vi "layout.vi"(0 "reference":refnum<class "StateNode.lvclass">, 1 "graph":refnum<class "Graph.lvclass">, 2 "graphics":refnum<class "Graphics.lvclass">, 3 "grid":refnum<class "Grid.lvclass">, 5 "error in (no error)":errorcluster) -> (14 "reference out":refnum<class "StateNode.lvclass">, 19 "error out":errorcluster)   [LabVIEW 2014, in "StateNode.lvclass"]
doc: "public void layout(Graph g, Graphics2D g2, Grid grid)"
uses:
  <resource>/Framework/Providers/Open_GDS/UML/StateNode_class/StateNode.lvclass
  <resource>/Framework/Providers/Open_GDS/UML/Graph_class/Graph.lvclass
  <resource>/Framework/Providers/Open_GDS/UML/Graphics_class/Graphics.lvclass
  <resource>/Framework/Providers/Open_GDS/UML/Grid_class/Grid.lvclass
  <resource>/Framework/Providers/Open_GDS/UML/General/Rectangle/Rectangle Rectangle2D.ctl
  <resource>/Framework/Providers/Open_GDS/UML/MultiLineString_class/MultiLineString.lvclass
  <resource>/Framework/Providers/Open_GDS/UML/RectangularNode_class/RectangularNode.lvclass
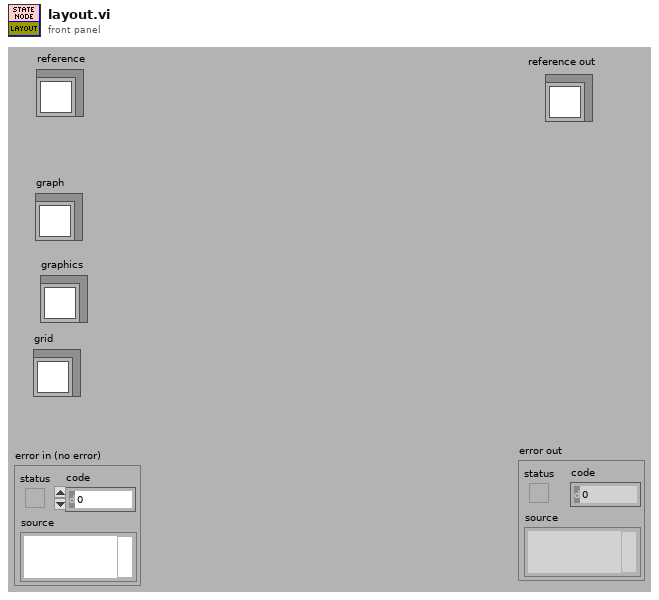
[diagram p1: front panel]
types:
  T1 = typedef "Rectangle Rectangle2D.ctl" = cluster{"x":dbl, "y":dbl, "width":dbl, "height":dbl}
  T2 = typedef "StateNode.lvclass/ObjectAttributes.ctl" = cluster{"state":refnum<class "MultiLineString.lvclass">, "action":refnum<class "MultiLineString.lvclass">, "DEFAULT_WIDTH":i32, "DEFAULT_HEIGHT":i32}
  T3 = typedef "RectangularNode.lvclass/ObjectAttributes.ctl" = cluster{"bounds":T1}
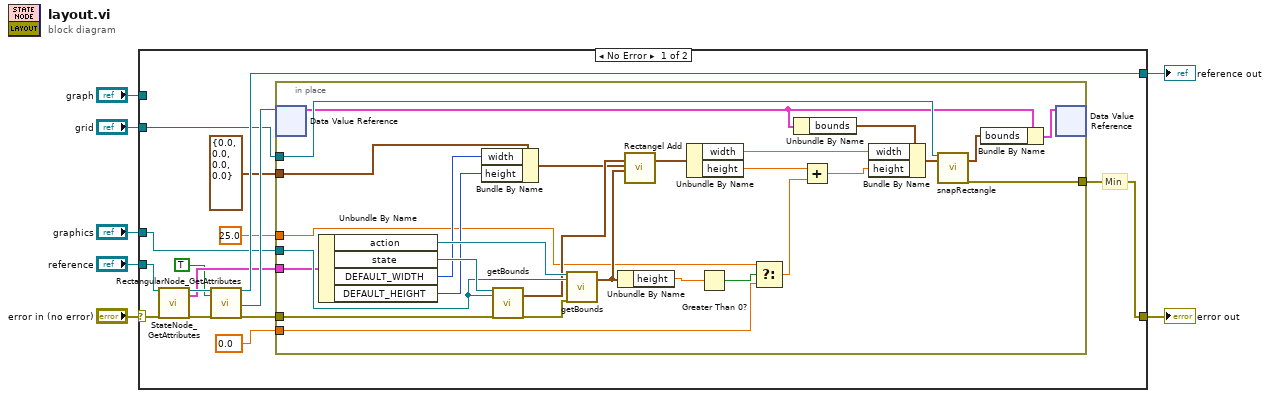
[diagram p0: block diagram]
diagram:
  n1 = case shown="No Error" "error in (no error)" {
    selector: "error in (no error)" -> [w20 w51]
    tunnel: "reference" -> [w22 w52]
    tunnel: [w10 w51] -> w6
    tunnel: [w21 w52] -> w5
    tunnel: "graph" -> [_ _]
    tunnel: "graphics" -> [w16 _]
    tunnel: "grid" -> [w11 _]
    frame No Error {
      # "Min"
      n2 = call <resource>:"StateNode_GetAttributes.vi"("reference in"=w22, "error in (no error)"=w20) -> ("reference out"=w19:refnum<class "StateNode.lvclass">, "Data"=w9:T2, "error out"=w18:errorcluster)  [unwired: 14 in, 1 out]
      n3 = call <resource>:"RectangularNode_GetAttributes.vi"("reference in"=w19, "OnlyGetDvrReference(False)"=TRUE, "error in (no error)"=w18) -> ("reference out"=w21:refnum<class "StateNode.lvclass">, "DataRef"=w17:refnum<data-value>, "error out"=w15:errorcluster)  [unwired: 13 in, 1 out]
      n4 = in-place {
        in-place-border: w16 -> [w44]
        in-place-border: w15 -> [w43]
        in-place-border: T1 {"x"=0.0, "y"=0.0, "width"=0.0, "height"=0.0} ("bounds") -> [w41]
        in-place-border: 0.0 ("x") -> [w30]
        in-place-border: 25.0 ("t") -> [w29]
        in-place-border: w11 -> [w28]
        in-place-border: [w26] -> w10
        in-place-border: w9 -> [w23]
        n5 = in-place-dvr #1(w17) -> (w25:T3)  [unwired: 1 out]
        n6 = Unbundle By Name(w23) -> ("action"=w50:refnum<class "MultiLineString.lvclass">, "state"=w49:refnum<class "MultiLineString.lvclass">, "DEFAULT_WIDTH"=w48:i32, "DEFAULT_HEIGHT"=w47:i32)
        n7 = Bundle By Name(cluster=w41, "width"=w48, "height"=w47) -> (w40:T1)
        n8 = call-dynamic "getBounds.vi"("reference"=w49, "graphics"=w44, "error in (no error)"=w43) -> ("bounds"=w42:T1, "error out"=w46:errorcluster)  [unwired: 15 out]
        n9 = call-dynamic "getBounds.vi"("reference"=w50, "graphics"=w44, "error in (no error)"=w46) -> ("bounds"=w45:T1)  [unwired: 16 out]
        n10 = Unbundle By Name(w45) -> ("height"=w38:dbl)
        n11 = call <resource>:"Rectangel Add.vi"("bounds1"=w42, "bounds2"=w40, "bounds3"=w45) -> ("boundsAdded"=w39:T1)  [unwired: 2 in, 14 out]
        n12 = Unbundle By Name(w39) -> ("width"=w37:dbl, "height"=w36:dbl)
        n13 = Greater Than 0?(x=w38) -> (x > 0?=w35:bool)
        n14 = Select(t=w29, s=w35, f=w30) -> (s? t:f=w31:dbl)
        n15 = Unbundle By Name(w25) -> ("bounds"=w34:T1)
        n16 = Add(x=w36, y=w31) -> (x+y=w33:dbl)
        n17 = Bundle By Name(cluster=w34, "width"=w37, "height"=w33) -> (w32:T1)
        n18 = call <resource>:"snapRectangle.vi"("reference"=w28, "bounds"=w32) -> ("boundsOut"=w27:T1, "error out"=w26:errorcluster)  [unwired: 1 in, 15 out]
        n19 = Bundle By Name(cluster=w25, "bounds"=w27) -> (w24:T3)
        n20 = in-place-dvr #1(w24) -> ()  [unwired: 2 out]
      }
    }
    frame Error {
    }
  }
  "reference out" <- w5
  "error out" <- w6
